vi "PID power calc.vi"(7 "DAQ state cluster in":T1={"DAQ state"=enum."Global comm", "device"="", "start (ms)"=0, "error"={"status"=FALSE, "code"=0, "source"=""}, "T cont"={"exec"={"T mode"=enum."Listening to exec", "exec setpoint"=0.0, "reset"=FALSE, "man power"=0.0, "man"=FALSE, "log"=FALSE, "clear"=FALSE}, "T status"={"Control status"=enum."In Settle Band", "Temp"=0.0, "Power"=0.0, "Time in settle band"=0.0, "Settled"=FALSE, "Low"=FALSE, "High"=FALSE, "Setpoint"=0.0, "Control"=FALSE, "In Settle Band"=FALSE}, "T params"={"Setpoint"=0.0, "Control Bandwidth"=0.0, "Integral Time"=0.0, "Int\nON"=FALSE, "Derivative Tme"=0.0, "Der\nON"=FALSE, "Settle Bandwidth"=0.0, "Settle Time"=0.0}, "utility"={"meas index"=0, "wait (ms)"=0, "H Vmax"=8.5, "power out"=5.0, "heat volt out"=0.0, "heat volt in"=0.0, "therm volt"=0.0, "t T P hist"=[], "cont hist"=[]}}} {"T cont"."utility"."therm volt" format="%_6g"; "T cont"."utility"."heat volt in" format="%_6g"; "T cont"."utility"."heat volt out" format="%_6g"; "T cont"."utility"."power out" format="%_6g"; "T cont"."utility"."H Vmax" format="%_6g"; "T cont"."exec"."man power" format="%_6g"; "T cont"."exec"."exec setpoint" format="%_6g"; "T cont"."T params"."Settle Time" step=1.0; "T cont"."T params"."Settle Bandwidth" step=0.01; "T cont"."T params"."Derivative Tme" step=0.01; "T cont"."T params"."Integral Time" step=1.0; "T cont"."T params"."Control Bandwidth" step=0.1; "T cont"."T params"."Setpoint" step=0.1; "T cont"."T status"."Setpoint" format="%_6g"; "T cont"."T status"."Power" format="%_6g"; "T cont"."T status"."Temp" format="%_6g"}) -> (8 "DAQ state cluster out":T1={"DAQ state"=enum."Global comm", "device"="", "start (ms)"=0, "error"={"status"=FALSE, "code"=0, "source"=""}, "T cont"={"exec"={"T mode"=enum."Listening to exec", "exec setpoint"=0.0, "reset"=FALSE, "man power"=0.0, "man"=FALSE, "log"=FALSE, "clear"=FALSE}, "T status"={"Control status"=enum."In Settle Band", "Temp"=0.0, "Power"=0.0, "Time in settle band"=0.0, "Settled"=FALSE, "Low"=FALSE, "High"=FALSE, "Setpoint"=0.0, "Control"=FALSE, "In Settle Band"=FALSE}, "T params"={"Setpoint"=0.0, "Control Bandwidth"=0.0, "Integral Time"=0.0, "Int\nON"=FALSE, "Derivative Tme"=0.0, "Der\nON"=FALSE, "Settle Bandwidth"=0.0, "Settle Time"=0.0}, "utility"={"meas index"=0, "wait (ms)"=0, "H Vmax"=8.5, "power out"=5.0, "heat volt out"=0.0, "heat volt in"=0.0, "therm volt"=0.0, "t T P hist"=[], "cont hist"=[]}}} {"T cont"."utility"."therm volt" format="%_6g"; "T cont"."utility"."heat volt in" format="%_6g"; "T cont"."utility"."heat volt out" format="%_6g"; "T cont"."utility"."power out" format="%_6g"; "T cont"."utility"."H Vmax" format="%_6g"; "T cont"."exec"."man power" format="%_6g"; "T cont"."exec"."exec setpoint" format="%_6g"; "T cont"."T params"."Settle Time" step=1.0; "T cont"."T params"."Settle Bandwidth" step=0.01; "T cont"."T params"."Derivative Tme" step=0.01; "T cont"."T params"."Integral Time" step=1.0; "T cont"."T params"."Control Bandwidth" step=0.1; "T cont"."T params"."Setpoint" step=0.1; "T cont"."T status"."Setpoint" format="%_6g"; "T cont"."T status"."Power" format="%_6g"; "T cont"."T status"."Temp" format="%_6g"})   [LabVIEW 2019]
doc: "This subVI is one of the states of the DAQ state machine in the bug experiment.\n\nThis state does a PID calulation to determine the power to output.\n\nIt proceeds to output power next.\n\nPaul K Dixon\nP3600\nCSUSB Physics"
uses:
  typedefs/DAQ T state cluster.ctl
  typedefs/DAQ T state enum.ctl
  typedefs/temp cont cluster.ctl
  typedefs/temp exec cluster.ctl
  typedefs/temp mode enum.ctl
  typedefs/temp indicator.ctl
  typedefs/temp control status.ctl
  typedefs/PID control parameters.ctl
  typedefs/temp cont utility.ctl
panel:
  out "in settle band":bool
  out "in control band":bool
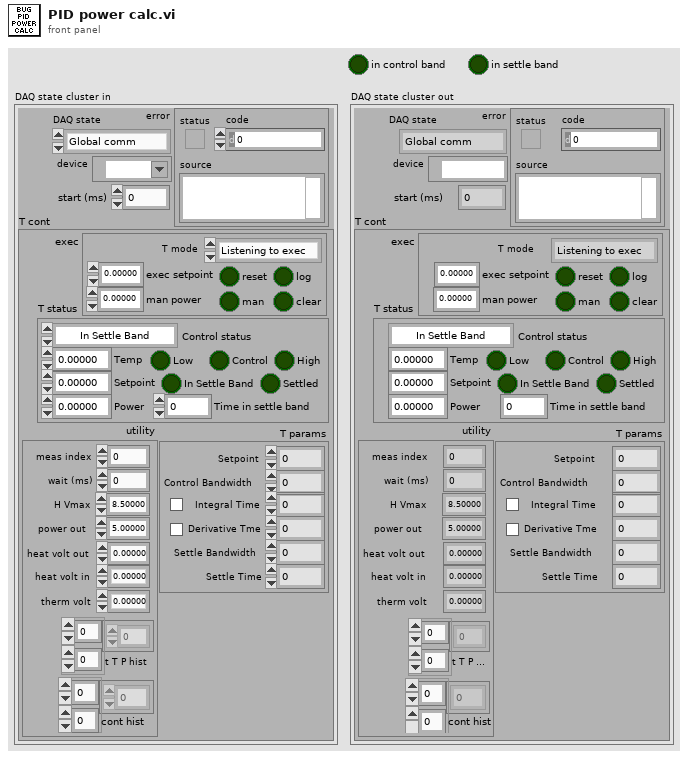
[diagram p1: front panel]
types:
  T1 = typedef "DAQ T state cluster.ctl" = cluster{"DAQ state":T2, "device":tag, "start (ms)":i32, "error":errorcluster, "T cont":T3}
  T2 = typedef "DAQ T state enum.ctl" = enum16{"Global comm", "Meas T & P", "PID power calc", "Man Power set", "Output Power", "Wait", "Exit"}
  T3 = typedef "temp cont cluster.ctl" = cluster{"exec":T4, "T status":T6, "T params":T8, "utility":T9}
  T4 = typedef "temp exec cluster.ctl" = cluster{"T mode":T5, "exec setpoint":dbl, "reset":bool, "man power":dbl, "man":bool, "log":bool, "clear":bool}
  T5 = typedef "temp mode enum.ctl" = enum16{"Setting up", "Listening to exec", "Exit"}
  T6 = typedef "temp indicator.ctl" = cluster{"Control status":T7, "Temp":dbl, "Power":dbl, "Time in settle band":dbl, "Settled":bool, "Low":bool, "High":bool, "Setpoint":dbl, "Control":bool, "In Settle Band":bool}
  T7 = typedef "temp control status.ctl" = enum16{"In Settle Band", "In Control Band", "Below Control Band", "Above Control Band"}
  T8 = typedef "PID control parameters.ctl" = cluster{"Setpoint":dbl, "Control Bandwidth":dbl, "Integral Time":dbl, "Int\nON":bool, "Derivative Tme":dbl, "Der\nON":bool, "Settle Bandwidth":dbl, "Settle Time":dbl}
  T9 = typedef "temp cont utility.ctl" = cluster{"meas index":i32, "wait (ms)":i32, "H Vmax":dbl, "power out":dbl, "heat volt out":dbl, "heat volt in":dbl, "therm volt":dbl, "t T P hist":dbl[][], "cont hist":dbl[][]}
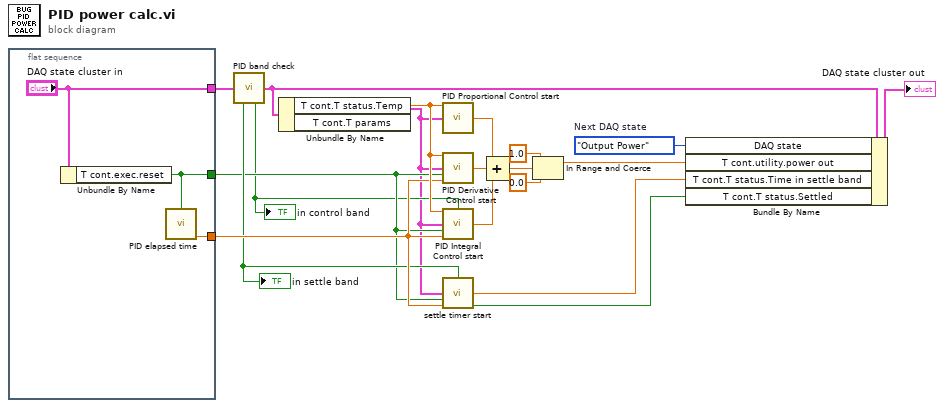
[diagram p0: block diagram]
diagram:
  w18 = DAQ_T_state_enum."Output Power"  # Next DAQ state
  n1 = flat-sequence {
    tunnel: [w22] -> w8
    tunnel: [w21] -> w6
    tunnel: ["DAQ state cluster in"] -> w1
    frame #0 {
      n2 = Unbundle By Name("DAQ state cluster in") -> ("T cont.exec.reset"=w21:bool)
      n3 = call "PID elapsed time.vi"("reset"=w21) -> ("elaspsed time (sec)"=w22:dbl)  [unwired: 13 in, 1 out]
    }
  }
  n4 = call "PID band check.vi"("DAQ state cluster in"=w1) -> ("DAQ state cluster out"=w17:T1, "In SB"=w7:bool, "In CB"=w5:bool)  [unwired: 12 in]
  "in control band" <- w5
  "in settle band" <- w7
  n5 = Unbundle By Name(w17) -> ("T cont.T status.Temp"=w9:dbl, "T cont.T params"=w2:T8)
  n6 = call "PID Proportional Control start.vi"("Temp"=w9, "Control Parameters"=w2) -> ("Proportional Power"=w15:dbl)  [unwired: 13 in]
  n7 = call "PID Derivative Control start.vi"("Temp In (deg C)"=w9, "Control Parameters"=w2, "reset"=w6, "delta t"=w8) -> ("Derivative Power"=w16:dbl)  [unwired: 11 in]
  n8 = call "PID Integral Control start.vi"("Temp In (deg C)"=w9, "in control band"=w5, "Control Parameters"=w2, "reset"=w6, "delta t"=w8) -> ("Integral Power"=w14:dbl)  [unwired: 10 in]
  n9 = call "settle timer start.vi"("in settle band"=w7, "Control Parameters"=w2, "reset"=w6, "delta t"=w8) -> ("time in settle band"=w4:dbl, "settled"=w3:bool)  [unwired: 10 in]
  n10 = Compound Arithmetic op=ADD(w15, w16, w14) -> (w13:dbl)
  n11 = In Range and Coerce(upper limit=1.0, x=w13, lower limit=0.0) -> (coerced(x)=w10:dbl)  [unwired: 1 out]
  n12 = Bundle By Name(cluster=w17, "DAQ state"=w18, "T cont.utility.power out"=w10, "T cont.T status.Time in settle band"=w4, "T cont.T status.Settled"=w3) -> (→"DAQ state cluster out":T1)
